vi "Update_SourceItem_from_Linker.vi"(8 "error in (no error)":errorcluster, 10 "linkerInfo":T2, 11 "AB_Source in":refnum<class "AB_Source.lvclass">) -> (0 "error out":errorcluster, 3 "AB_Source out":refnum<class "AB_Source.lvclass">)   [LabVIEW 2020, in "AB_Source.lvclass"]
uses:
  <vilib>/AppBuilder/AB_Classes/Source/AB_Source.lvclass
  <vilib>/Utility/lvfile.llb/LVFileType.ctl
  <vilib>/AppBuilder/AB_Classes/Source/AB_Source.lvclass/AB_Source.ctl
  <vilib>/Utility/lvfile.llb/NI_FileType.lvlib
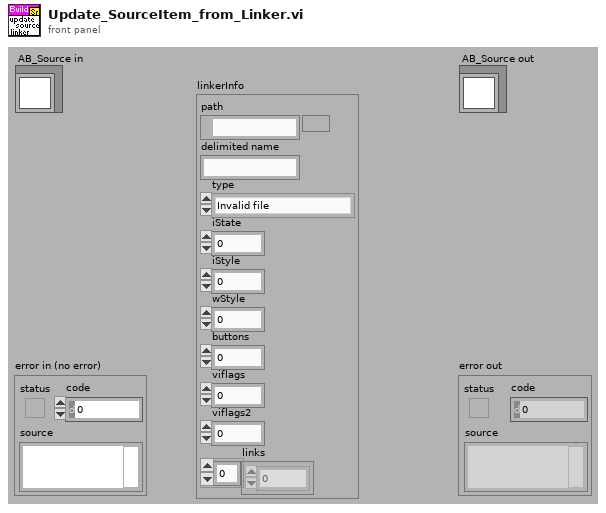
[diagram p1: front panel]
types:
  T1 = typedef "NI_FileType.lvlib/LVFileType.ctl" = enum32{"Invalid file", "Unknown type", "Instrument", "Control", "Polymorphic VI", "Project", "Library", "LVClass", "XControl", "XNode", "Shared library", ".NET assembly", "ActiveX interface", "CIN", "Run-time menu", "Palette menu", "Help file", "LLB", "XNode Edit Dependency", "Class Private Data Control", "Statechart", "MathScript .m file", "Ladder Diagram", "LVLibp", "XNode Build Dependency"}
  T2 = cluster{"path":path, "delimited name":string, "type":T1, "iState":u32, "iStyle":u16, "wStyle":u16, "buttons":u16, "viflags":u32, "viflags2":u32, "links":u32[]}
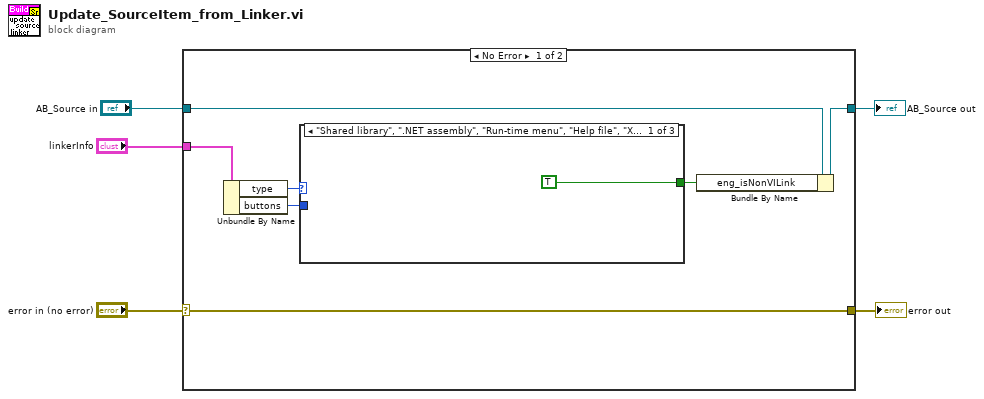
[diagram p0: block diagram]
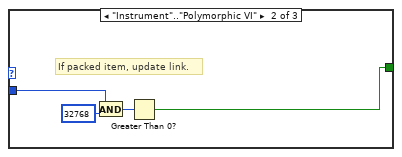
[diagram p2: hidden frame]
diagram:
  n1 = case shown="No Error" "error in (no error)" {
    selector: "error in (no error)" -> [w12 w19]
    tunnel: [w12 w19] -> w4
    tunnel: [w10 w18] -> w2
    tunnel: "AB_Source in" -> [w11 w18]
    tunnel: "linkerInfo" -> [w9 _]
    frame No Error {
      n2 = Unbundle By Name(w9) -> ("type"=w8:T1, "buttons"=w6:u16)
      n3 = case shown="\"Shared library\", \".NET assembly\", \"Run-time menu\", \"Help file\", \"XNode Edit Dependency\", \"MathScript .m file\", \"XNode Build Dependency\"" w8 {
        tunnel: [TRUE w14 _] -> w7
        tunnel: w6 -> [_ w15 _]
        frame "Shared library", ".NET assembly", "Run-time menu", "Help file", "XNode Edit Dependency", "MathScript .m file", "XNode Build Dependency" {
        }
        frame "Instrument".."Polymorphic VI" {
          # "If packed item, update link."
          n4 = And(x=w15, y=u16 32768) -> (x .and. y?=w16:u16)
          n5 = Greater Than 0?(x=w16) -> (x > 0?=w14:bool)
        }
        frame Default {
        }
      }
      n6 = Bundle By Name(cluster=w11, "eng_isNonVILink"=w7) -> (w10:refnum<class "AB_Source.lvclass">)
    }
    frame Error {
    }
  }
  "error out" <- w4
  "AB_Source out" <- w2
